vi "Calculate Termination.vi"(4 "Port (Port 1)":u16(ring) items=["Port 1", "Port 2"], 5 "Gamma":cdb[](array[numeric]), 6 "error in (no error)":errorcluster, 9 "2-port S-parameters":cdb[][](array[numeric])) -> (0 "error out":errorcluster, 3 "Termination":cdb[](array[numeric]))   [LabVIEW 2023, in "NI_HFNetworkAnalysis.lvlib"]
doc: "Calculates the reflection factor of the termination, for different frequencies, at the specified port of a 2-port network while the other port presents the specified input impedance. \n\nThe network is described by 2-port S-parameters <b>(S11,S12,S21,S22)</b> at different frequencies and the input impednace is described by its reflection factor at those frequencies.\n\n<b>Known Limitations</b>\nOnly 2-port networks are supported."
uses:
  NI_HFNetworkAnalysis.lvlib
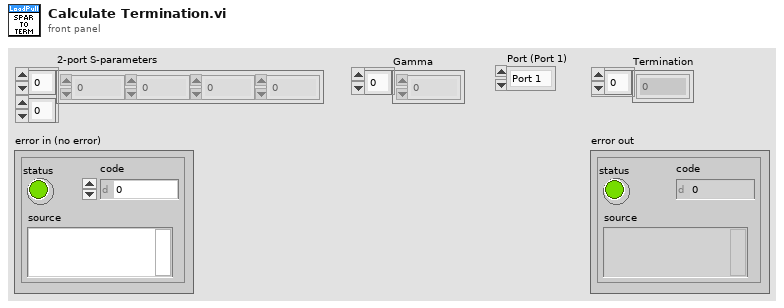
[diagram p1: front panel]
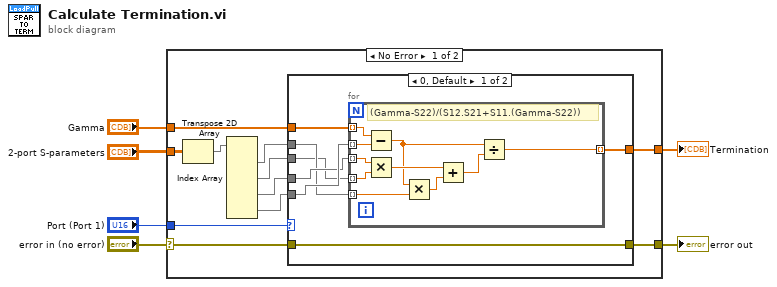
[diagram p0: block diagram]
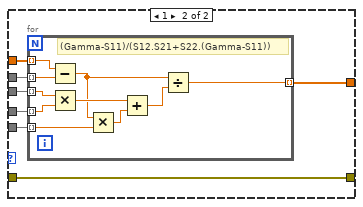
[diagram p2: hidden frame]
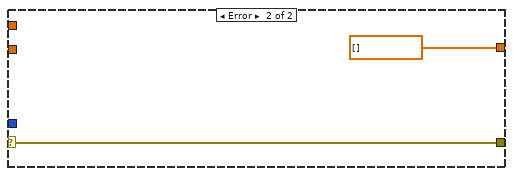
[diagram p3: hidden frame]
diagram:
  n1 = case shown="No Error" "error in (no error)" {
    selector: "error in (no error)" -> [w9 w53]
    tunnel: "Gamma" -> [w17 _]
    tunnel: [w16 cdb[] []] -> w5
    tunnel: "2-port S-parameters" -> [w15 _]
    tunnel: "Port (Port 1)" -> [w11 _]
    tunnel: [w10 w53] -> w2
    frame No Error {
      n2 = Transpose 2D Array(2D array=w15) -> (transposed array=w14:cdb[][])
      n3 = Index Array(array=w14) -> (element #1=w13:cdb[], element #2=w7:cdb[], element #3=w8:cdb[], element #4=w12:cdb[])  [unwired: 8 in]
      n4 = case shown="0, Default" w11 {
        tunnel: w17 -> [w24 w41]
        tunnel: [w19 w36] -> w16
        tunnel: w13 -> [w20 w40]
        tunnel: w8 -> [w22 w39]
        tunnel: w12 -> [w23 w38]
        tunnel: [w21 w37] -> w10
        tunnel: w9 -> [w21 w37]
        tunnel: w7 -> [w18 w35]
        frame 0, Default {
          n5 = for {
            tunnel: w23 -> [w29] mode=indexing
            tunnel: w22 -> [w27] mode=indexing
            tunnel: w18 -> [w26] mode=indexing
            tunnel: w20 -> [w25] mode=indexing
            tunnel: w24 -> [w30] mode=indexing
            tunnel: [w28] -> w19 mode=indexing
            # "(Gamma-S22)/(S12.S21+S11.(Gamma-S22))"
            n6 = Subtract(x=w30, y=w29) -> (x-y=w31:cdb)
            n7 = Multiply(x=w27, y=w26) -> (x*y=w33:cdb)
            n8 = Multiply(x=w31, y=w25) -> (x*y=w34:cdb)
            n9 = Add(x=w33, y=w34) -> (x+y=w32:cdb)
            n10 = Divide(x=w31, y=w32) -> (x/y=w28:cdb)
          }
        }
        frame 1 {
          n11 = for {
            tunnel: w40 -> [w51] mode=indexing
            tunnel: w35 -> [w48] mode=indexing
            tunnel: w39 -> [w49] mode=indexing
            tunnel: w38 -> [w47] mode=indexing
            tunnel: w41 -> [w50] mode=indexing
            tunnel: [w42] -> w36 mode=indexing
            # "(Gamma-S11)/(S12.S21+S22.(Gamma-S11))"
            n12 = Subtract(x=w50, y=w51) -> (x-y=w43:cdb)
            n13 = Multiply(x=w48, y=w49) -> (x*y=w45:cdb)
            n14 = Multiply(x=w43, y=w47) -> (x*y=w46:cdb)
            n15 = Add(x=w45, y=w46) -> (x+y=w44:cdb)
            n16 = Divide(x=w43, y=w44) -> (x/y=w42:cdb)
          }
        }
      }
    }
    frame Error {
    }
  }
  "Termination" <- w5
  "error out" <- w2
